vi "Vision Data.vi"() -> (0 "Dis":bool, 1 "S?":bool, 2 "S Dir":bool)   [LabVIEW 2016]
uses:
  Robot Global Data.vi
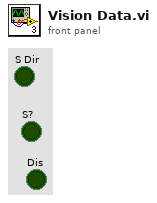
[diagram p1: front panel]
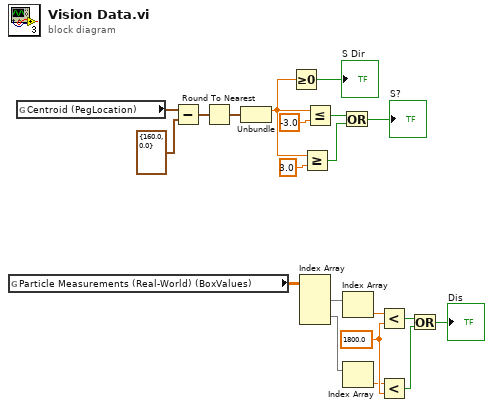
[diagram p0: block diagram]
diagram:
  w8 = 1800.0
  n1 = global read "Robot Global Data.vi" "Particle Measurements (Real-World) (BoxValues)"() -> (w11:dbl[][])
  n2 = global read "Robot Global Data.vi" "Centroid (PegLocation)"() -> (w14:cluster{"X Centroid":sgl, "Y Centroid":sgl})
  n3 = Subtract(x=w14, y=cluster{"X Centroid":sgl, "Y Centroid":sgl} {"X Centroid"=160.0, "Y Centroid"=0.0}) -> (x-y=w15:cluster{"X Centroid":sgl, "Y Centroid":sgl})
  n4 = Round To Nearest(number=w15) -> (nearest integer value=w20:cluster{"X Centroid":sgl, "Y Centroid":sgl})
  n5 = Unbundle(w20) -> ("X Centroid"=w12:sgl)  [unwired: 1 out]
  n6 = Greater Or Equal To 0?(x=w12) -> (x >= 0?=→"S Dir":bool)
  n7 = Index Array(array=w11) -> (element #1=w10:dbl[], element #2=w9:dbl[])  [unwired: 4 in]
  n8 = Greater Or Equal?(x=w12, y=sgl 3.0) -> (x >= y?=w18:bool)
  n9 = Less Or Equal?(x=w12, y=sgl -3.0 ("x")) -> (x <= y?=w19:bool)
  n10 = Or(x=w19, y=w18) -> (x .or. y?=→"S?":bool)
  n11 = Index Array(array=w10) -> (element=w5:dbl)  [unwired: 1 in]
  n12 = Index Array(array=w9) -> (element=w4:dbl)  [unwired: 1 in]
  n13 = Less?(x=w5, y=w8) -> (x < y?=w7:bool)
  n14 = Less?(x=w4, y=w8) -> (x < y?=w6:bool)
  n15 = Or(x=w7, y=w6) -> (x .or. y?=→"Dis":bool)
